vi "Increase NOK Counter.vi"(8 "error in (no error)":errorcluster) -> (0 "error out":errorcluster)   [LabVIEW 2023, in "Counters.lvlib"]
uses:
  Counters.lvlib
  <vilib>/Utility/config.llb/Read Key (U32).vi
  <vilib>/Utility/config.llb/Write Key (U32).vi
  <vilib>/Utility/config.llb/NI_LVConfig.lvlib
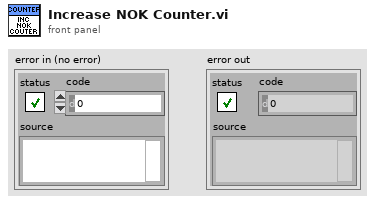
[diagram p1: front panel]
types:
  T1 = typedef "NI_LVConfig.lvlib/Config Data RefNum.ctl" = refnum<k1>
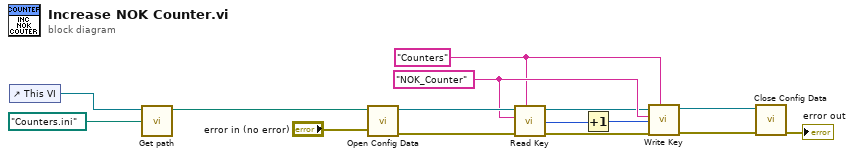
[diagram p0: block diagram]
diagram:
  w9 = "NOK_Counter" ("key")
  w8 = "Counters" ("section")
  n1 = control-ref of="This VI"() -> (w2:refnum<vi>)
  n2 = call "Get path.vi"("File mame"=path "Counters.ini" ("configuration file path"), "VI in"=w2) -> ("File path"=w1:path)  [unwired: 9 in]
  n3 = call <vilib>:"Open Config Data.vi"("error in (no error)"="error in (no error)", "configuration file path"=w1) -> ("error out"=w12:errorcluster, "refnum"=w13:T1)  [unwired: 7 in, 1 out]
  n4 = call-poly <vilib>:"Read Key.vi"("section"=w8, "error in (no error)"=w12, "key"=w9, "refnum"=w13) -> ("error out"=w5:errorcluster, "value"=w11:u32, "refnum out"=w4:T1)  [unwired: 4 in, 1 out]
  n5 = Increment(x=w11) -> (x+1=w10:u32)
  n6 = call-poly <vilib>:"Write Key.vi"("section"=w8, "error in (no error)"=w5, "value"=w10, "key"=w9, "refnum"=w4) -> ("error out"=w6:errorcluster, "refnum out"=w7:T1)  [unwired: 4 in, 1 out]
  n7 = call <vilib>:"Close Config Data.vi"("error in (no error)"=w6, "refnum"=w7) -> ("error out"=→"error out":errorcluster)  [unwired: 8 in, 1 out]
